vi "Release Gum.vi"(0 "reference in":refnum<class "Gum Machine.lvclass">, 5 "error in (no error)":errorcluster) -> (14 "reference out":refnum<class "Gum Machine.lvclass">, 19 "error out":errorcluster)   [LabVIEW 2013, in "Gum Machine.lvclass"]
uses:
  Gum Machine.lvclass
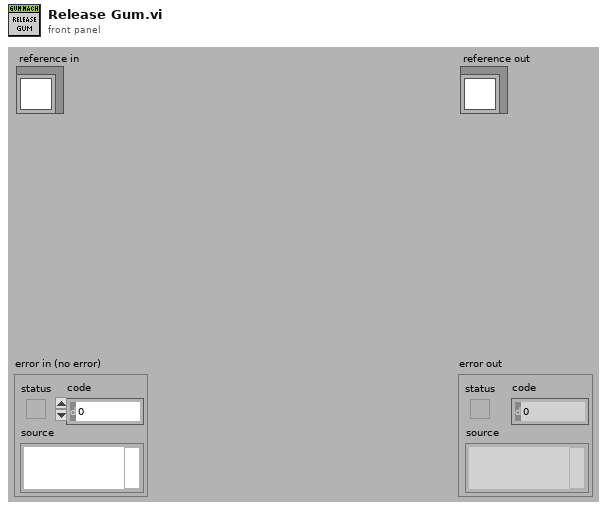
[diagram p1: front panel]
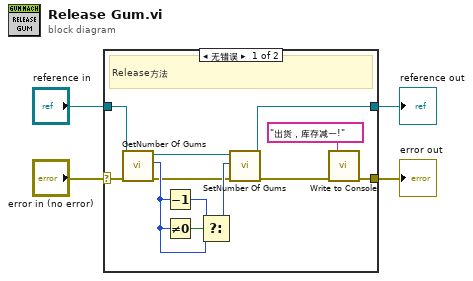
[diagram p0: block diagram]
diagram:
  n1 = case shown="无错误" "error in (no error)" {
    selector: "error in (no error)" -> [w14 w18]
    tunnel: [w6 w18] -> w3
    tunnel: [w8 w17] -> w1
    tunnel: "reference in" -> [w16 w17]
    frame No Error {
      # "Release方法"
      n2 = call-dynamic "GetNumber Of Gums.vi"("error in (no error)"=w14, "reference in"=w16) -> ("error out"=w9:errorcluster, "Number Of Gums"=w11:u32, "reference out"=w15:refnum<class "Gum Machine.lvclass">)  [unwired: 7 in]
      n3 = Decrement(x=w11) -> (x-1=w12:u32)
      n4 = Not Equal To 0?(x=w11) -> (x != 0?=w13:bool)
      n5 = Select(t=w12, s=w13, f=w11) -> (s? t:f=w10:u32)
      n6 = call-dynamic "SetNumber Of Gums.vi"("error in (no error)"=w9, "Number Of Gums"=w10, "reference in"=w15) -> ("error out"=w7:errorcluster, "reference out"=w8:refnum<class "Gum Machine.lvclass">)  [unwired: 7 in]
      n7 = call "Write to Console.vi"("error in (no error)"=w7, "Input"="出货，库存减一!") -> ("error out"=w6:errorcluster)  [unwired: 9 in]
    }
    frame Error {
    }
  }
  "error out" <- w3
  "reference out" <- w1
